vi "VCS Get Sensor Type.vi"(8 "error in (no error)":errorcluster, 11 "axis in":cluster{"keyHandle":u32, "nodeId":u16}={"keyHandle"=0, "nodeId"=1}) -> (0 "error out":errorcluster, 1 "sensorType":u16(ring) items=["Unknown sensor", "Incremental encoder with index (3-channel)", "Incremental encoder without index (2-channel)", "Hall sensors", "SSI encoder binary coded", "SSI encoder grey coded"], 3 "axis out":cluster{"keyHandle":u32, "nodeId":u16}={"keyHandle"=0, "nodeId"=1})   [LabVIEW 2018]
doc: "With function <B>VCS_GetSensorType</B> it is possible to read the sensor type."
uses:
  Resources/EposCmd.dll
  Resources/EposCmd64.dll
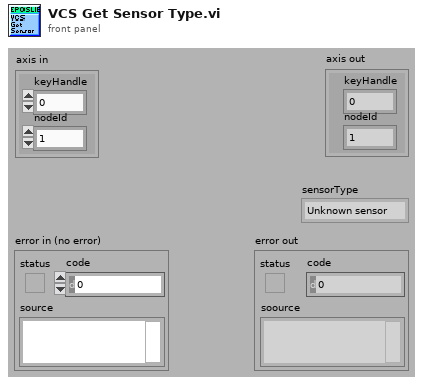
[diagram p1: front panel]
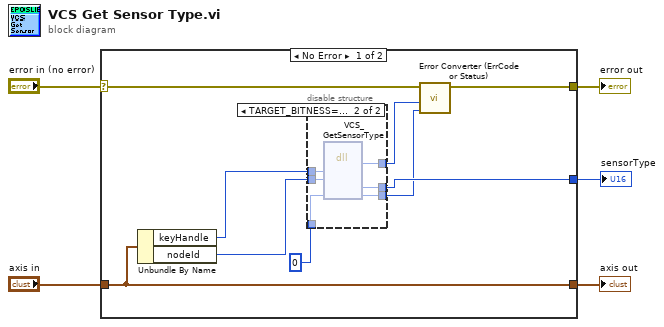
[diagram p0: block diagram]
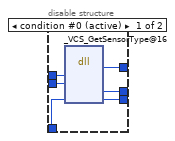
[diagram p2: hidden frame]
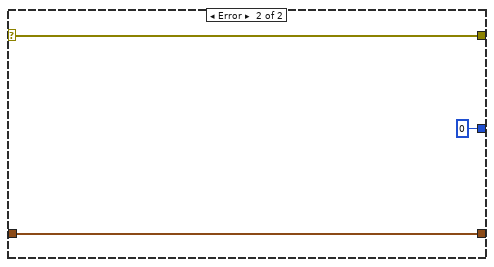
[diagram p3: hidden frame]
diagram:
  n1 = case shown="No Error" "error in (no error)" {
    selector: "error in (no error)" -> [w12 w28]
    tunnel: "axis in" -> [w14 w29]
    tunnel: [w14 w29] -> w4
    tunnel: [w13 w28] -> w3
    tunnel: [w11 u16 0 ("pSensorType")] -> w1
    frame No Error {
      n2 = Unbundle By Name(w14) -> ("keyHandle"=w9:u32, "nodeId"=w8:u16)
      n3 = disable-structure shown="TARGET_BITNESS==64" {
        disable-tunnel: [w20 w26] -> w11
        disable-tunnel: u32 0 ("pErrorCode") -> [w19 w25]
        disable-tunnel: w9 -> [w18 w24]
        disable-tunnel: w8 -> [w17 w23]
        disable-tunnel: [w16 w22] -> w7
        disable-tunnel: [w15 w21] -> w6
        frame condition #0 (active) {
          n4 = dll-call lib="C:/Projeto em LabVIEW/EPOS-LabVIEW-Instrument-Driver-En/LabVIEW/maxon EPOS/Resources/EposCmd.*" fn="_VCS_GetSensorType@16"("KeyHandle"=w18, "NodeId"=w17, "pErrorCode"=w19) -> (w16:i32, "pSensorType"=w20:u16, "pErrorCode"=w15:u32)  [unwired: 6 in, 2 out]
        }
        frame condition #1 {
          n5 = dll-call lib="C:/setup/Resources/EposCmd64.*" fn="VCS_GetSensorType" ("EposCmd.dll:_VCS_GetSensorType@16")("KeyHandle"=w24, "NodeId"=w23, "pErrorCode"=w25) -> ("Rückgabetyp"=w22:i32, "pSensorType"=w26:u16, "pErrorCode"=w21:u32)  [unwired: 6 in, 2 out]
        }
      }
      n6 = call "Error Converter (ErrCode or Status).vi"("error code"=w6, "return type"=w7, "error in (no error)"=w12) -> ("error out"=w13:errorcluster)  [unwired: 7 in]
    }
    frame Error {
    }
  }
  "sensorType" <- w1
  "error out" <- w3
  "axis out" <- w4
